vi "Write Ref TC and Order.vi"(8 "error in (no error)":errorcluster, 9 "order":i32, 10 "TC (s)":dbl, 11 "Lockin.DAQ":refnum<class "Lockin.DAQ.lvclass">) -> (0 "error out":errorcluster, 3 "Lockin.DAQ out":refnum<class "Lockin.DAQ.lvclass">)   [LabVIEW 2016, in "Lockin.DAQ.lvclass"]
uses:
  Lockin.DAQ.lvclass
  Lockin.DAQ.lvclass/Lockin.DAQ.ctl
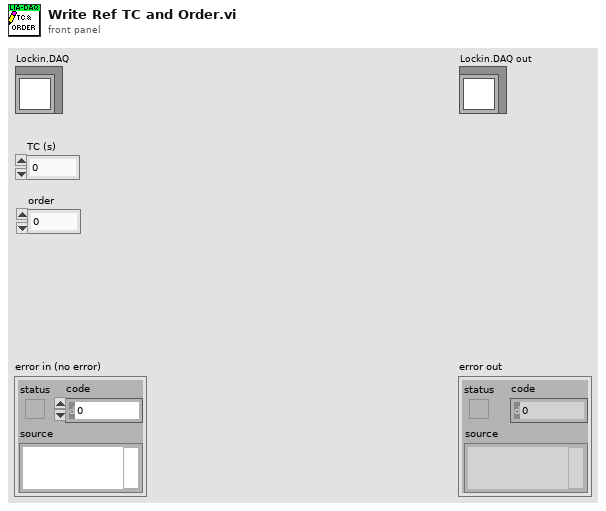
[diagram p1: front panel]
types:
  T1 = typedef "Lockin.DAQ.lvclass/REF-cluster.ctl" = T2[]
  T2 = typedef "Instrument.Lockin.UI.lvclass/REF Channel--Cluster.ctl" = cluster{"Enable?":bool, "Channel":i32, "Frequency":dbl, "Phase":dbl, "TC":dbl, "Order":i32}
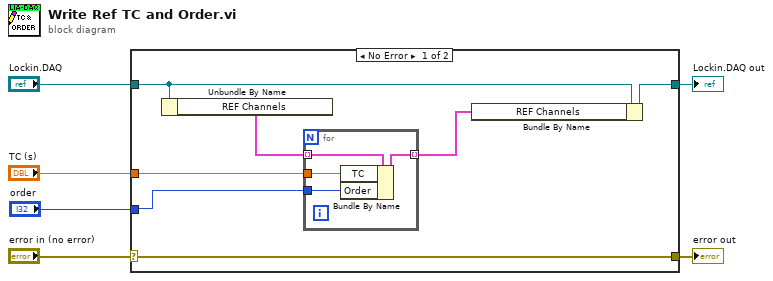
[diagram p0: block diagram]
diagram:
  n1 = case shown="No Error" "error in (no error)" {
    selector: "error in (no error)" -> [w13 w18]
    tunnel: [w13 w18] -> w5
    tunnel: [w9 w19] -> w3
    tunnel: "Lockin.DAQ" -> [w10 w19]
    tunnel: "TC (s)" -> [w12 _]
    tunnel: "order" -> [w11 _]
    frame No Error {
      n2 = Unbundle By Name(w10) -> ("REF Channels"=w7:T1)
      n3 = for {
        tunnel: w12 -> [w17]
        tunnel: w11 -> [w16]
        tunnel: w7 -> [w15] mode=indexing
        tunnel: [w14] -> w8 mode=indexing
        n4 = Bundle By Name(cluster=w15, "TC"=w17, "Order"=w16) -> (w14:T2)
      }
      n5 = Bundle By Name(cluster=w10, "REF Channels"=w8) -> (w9:refnum<class "Lockin.DAQ.lvclass">)
    }
    frame Error {
    }
  }
  "error out" <- w5
  "Lockin.DAQ out" <- w3
